vi "ReadTempSense.vi"(0 "COMPORT":refnum<visa-resource-name>="COM4", 11 "error in (no error)":errorcluster, 13 "Open/Close Serial":bool) -> (3 "tmon(str)":string, 4 "comport":refnum<visa-resource-name>="COM4", 8 "temp(c)":dbl[](array[numeric]), 15 "error out":errorcluster)   [LabVIEW 2018]
panel:
  out "All Success":bool=TRUE
  out "output 2":string
  out "string":string="\r\n"
  out "Success":bool[](array[boolean])=[TRUE]
  in  "Command ( ; seperation)":string="rd tmon"
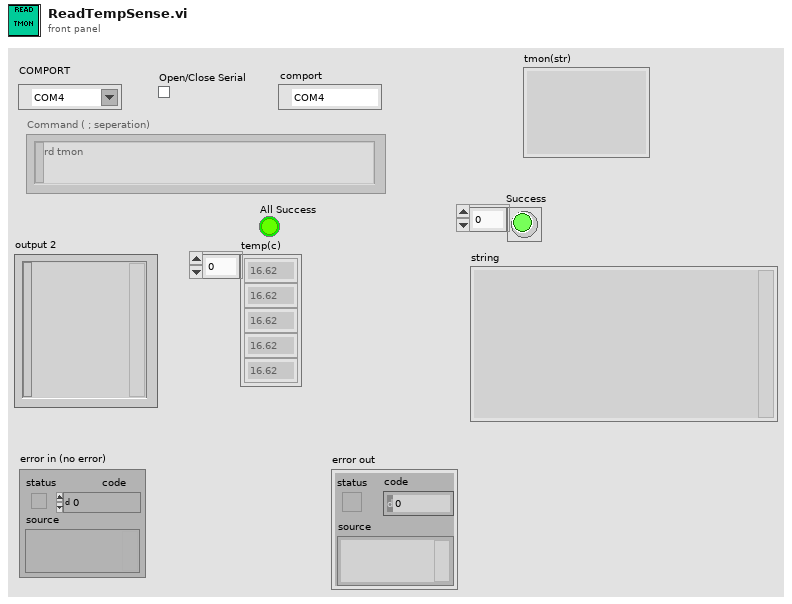
[diagram p1: front panel]
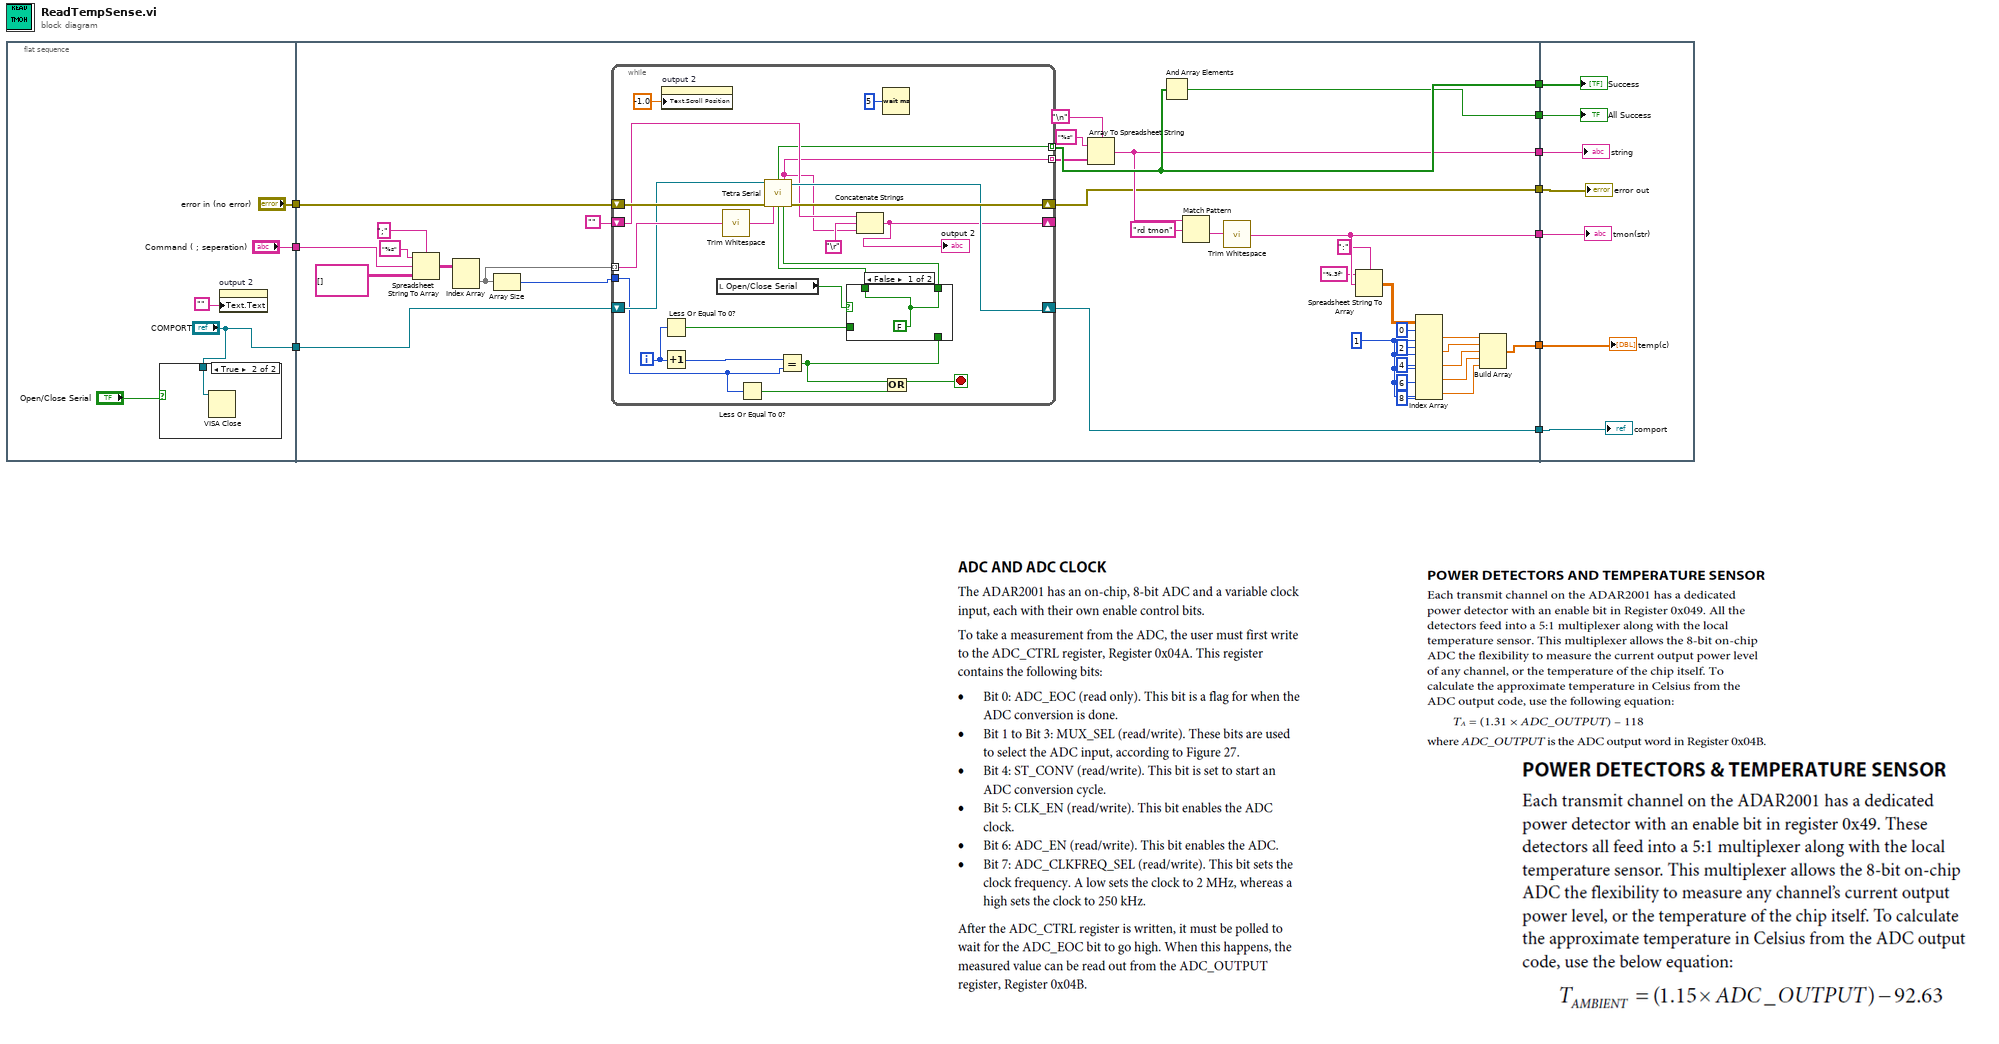
[diagram p0: block diagram]
diagram:
  n1 = flat-sequence {
    tunnel: ["error in (no error)"] -> w10
    tunnel: ["COMPORT"] -> w9
    tunnel: ["Command ( ; seperation)"] -> w8
    tunnel: w10 -> [w48]
    tunnel: w9 -> [w35]
    tunnel: w8 -> [w44]
    tunnel: [w42] -> w7
    tunnel: [w41] -> w6
    tunnel: [w32] -> w5
    tunnel: [w37] -> w4
    tunnel: [w36] -> w3
    tunnel: [w34] -> w2
    tunnel: [w17] -> w1
    tunnel: w7 -> [w80]
    tunnel: w6 -> [w81]
    tunnel: w5 -> [w82]
    tunnel: w4 -> [w83]
    tunnel: w3 -> [w84]
    tunnel: w2 -> [w85]
    tunnel: w1 -> [w79]
    frame #0 {
      n2 = case shown="True" "Open/Close Serial" {
        tunnel: "COMPORT" -> [_ w16]
        frame False {
        }
        frame True {
          n3 = VISA Close(VISA resource name=w16) -> ()  [unwired: 1 in, 1 out]
        }
      }
      n4 = property on="output 2" class="Str"("Text.Text"="") -> ()  [unwired: 2 in, 2 out]
    }
    frame #1 {
      w28 = 1 ("disabled index (col)")
      n5 = Spreadsheet String To Array(delimiter (Tab)=";", format string="%s", spreadsheet string=w44, array type (2D Dbl)=string[][] []) -> (array=w49:string[][])
      n6 = Index Array(array=w49) -> (element=w47:string[])  [unwired: 2 in]
      n7 = Array Size(array=w47) -> (size(s)=w39:i32)
      n8 = while {
        shift-right: [w75] -> w34
        shift-left: w48 -> [w74]
        shift-right: [w73] -> w37
        shift-left: w35 -> [w62]
        tunnel: [w68] -> w40 mode=indexing
        tunnel: w47 -> [w72] mode=indexing
        tunnel: w39 -> [w60]
        shift-right: [w65] -> _
        shift-left: "" -> [w69]
        tunnel: [w66] -> w42 mode=indexing
        i -> [w63]
        stop <- w61 stop-if-true
        n9 = property on="output 2" class="Str"("Text.Scroll Position"=-1.0) -> ()  [unwired: 2 in, 2 out]
        n10 = Less Or Equal To 0?(x=w63) -> (x <= 0?=w56:bool)
        n11 = Increment(x=w63) -> (x+1=w64:i32)
        n12 = local read "Open/Close Serial"() -> (w53:bool)
        n13 = call <vilib>:"Trim Whitespace.vi"("string"=w72) -> ("trimmed string"=w67:string)  [unwired: 1 in]
        n14 = Less Or Equal To 0?(x=w60) -> (x <= 0?=w59:bool)
        n15 = Equal?(x=w64, y=w60) -> (x = y?=w54:bool)
        n16 = case shown="False" w53 {
          tunnel: [w76 w78] -> w57
          tunnel: w56 -> [_ w78]
          tunnel: [w76 w77] -> w55
          tunnel: w54 -> [_ w77]
          frame False {
            w76 = FALSE
          }
          frame True {
          }
        }
        n17 = call "Tetra Serial.vi"("COMPORT"=w62, "error in (no error)"=w74, "Command"=w67, "Open Ser(t)"=w57, "Close Ser(t)"=w55) -> ("Success"=w66:bool, "output"=w68:string, "comport"=w73:refnum<visa-resource-name>, "error out"=w75:errorcluster)  [unwired: 6 in, 1 out]
        n18 = Concatenate Strings(w69, "\r", w68) -> (w65:string)
        "output 2" <- w65
        n19 = Wait (ms)(milliseconds to wait=u32 5) -> ()  [unwired: 1 out]
        n20 = Or(x=w54, y=w59) -> (x .or. y?=w61:bool)
      }
      n21 = Array To Spreadsheet String(delimiter (Tab)="\n", array=w40, 3:"%s" ("format string")) -> (spreadsheet string=w36:string)
      n22 = And Array Elements(Boolean array=w42) -> (logical AND=w41:bool)
      n23 = Match Pattern(string=w36, regular expression="rd tmon") -> (after substring=w33:string)  [unwired: 1 in, 3 out]
      n24 = call <vilib>:"Trim Whitespace.vi"("string"=w33) -> ("trimmed string"=w32:string)  [unwired: 1 in]
      n25 = Spreadsheet String To Array(delimiter (Tab)=":", format string="%.3f", spreadsheet string=w32) -> (array=w29:dbl[][])  [unwired: 1 in]
      n26 = Index Array(array=w29, index (row) #1=0 ("disabled index (row)"), index (col) #1=w28, index (row) #2=2 ("disabled index (row)"), index (col) #2=w28, index (row) #3=4 ("disabled index (row)"), index (col) #3=w28, index (row) #4=6 ("disabled index (row)"), index (col) #4=w28, index (row) #5=8 ("disabled index (row)"), index (col) #5=w28) -> (element #1=w22:dbl, element #2=w21:dbl, element #3=w20:dbl, element #4=w19:dbl, element #5=w18:dbl)
      n27 = Build Array(w22, w21, w20, w19, w18) -> (w17:dbl[])
    }
    frame #2 {
      "Success" <- w80
      "All Success" <- w81
      "tmon(str)" <- w82
      "temp(c)" <- w79
      "comport" <- w83
      "string" <- w84
      "error out" <- w85
    }
  }
